vi "Send Configure Acquisition Record.vi"(6 "acquisition start time (0.0 s)":dbl[unit] format="%.3f", 7 "Message Priority (Normal)":T1=enum."Normal", 8 "error in (no error)":errorcluster, 9 "min record length (100 samples)":i32=100, 10 "time per record (1.0E-3 s)":dbl[unit]=0.001 format="%^.2e", 11 "Message Enqueuer":refnum<class "Message Enqueuer.lvclass">) -> (0 "error out":errorcluster, 3 "Message Enqueuer out":refnum<class "Message Enqueuer.lvclass">)   [LabVIEW 2015, in "CS++Scope.lvlib" / "Configure Acquisition Record Msg.lvclass"]
doc: "Sends the <B>CS++Scope.lvlib:Configure Acquisition Record Msg.lvclass</B> message.\n\n<B>CS++Scope.lvlib:CS++Scope.lvclass:Configure Acquisition Record.vi</B> Description:\n\nThis VI configures the most commonly configured properties of the oscilloscope acquisition subsystem. These properties are the time per record, minimum record length, and the acquisition start time."
uses:
  Configure Acquisition Record Msg.lvclass
  <vilib>/ActorFramework/Message Enqueuer/Message Enqueuer.lvclass
  <vilib>/ActorFramework/Message Enqueuer/Message Priority.ctl
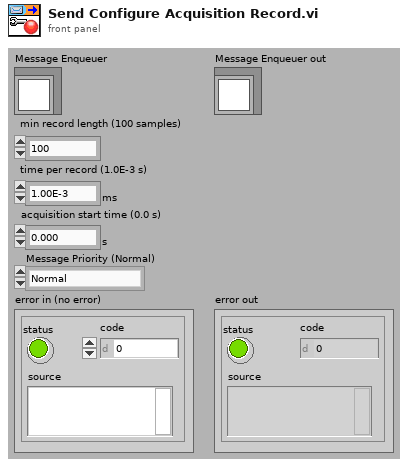
[diagram p1: front panel]
types:
  T1 = typedef "Actor Framework.lvlib/Message Enqueuer.lvclass/Message Priority.ctl" = enum16{"Low", "Normal", "High"}
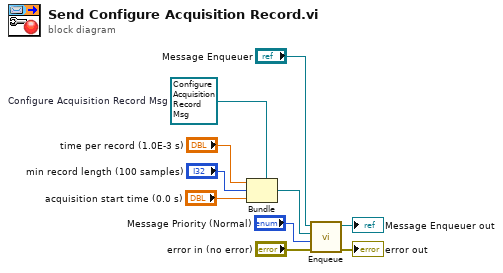
[diagram p0: block diagram]
diagram:
  w4 = refnum<class "Configure Acquisition Record Msg.lvclass"> refnum  # Configure Acquisition Record Msg
  n1 = Bundle(cluster=w4, "time per record (1.0E-3 s)", "min record length (100 samples)", "acquisition start time (0.0 s)") -> (w7:refnum<class "Configure Acquisition Record Msg.lvclass">)
  n2 = call <vilib>:"Enqueue.vi"("error in (no error)"="error in (no error)", "Message Priority (Normal)"="Message Priority (Normal)", "Message"=w7, "Message Enqueuer in"="Message Enqueuer") -> ("error out"=→"error out":errorcluster, "Message Enqueuer out"=→"Message Enqueuer out":refnum<class "Message Enqueuer.lvclass">)  [unwired: 6 in]
